vi "Nelson_Find_Whale_Color_Updated_Again.vi"(3 "error in":errorcluster, 5 "Image In":T1(plugin-control)) -> (0 "error out":errorcluster, 1 "Calibrated Centroid (Centroid 1)":cluster{"X Centroid":sgl, "Y Centroid":sgl} {"Y Centroid" format="%.2f"; "X Centroid" format="%.2f"}, 2 "Image Out":T1(plugin-control))   [LabVIEW 2014]
uses:
  <vilib>/vision/NI_Vision_Development_Module.lvlib
panel:
  out "Centroid (Centroid 1)":cluster{"X Centroid":sgl, "Y Centroid":sgl} {"Y Centroid" format="%.2f"; "X Centroid" format="%.2f"}
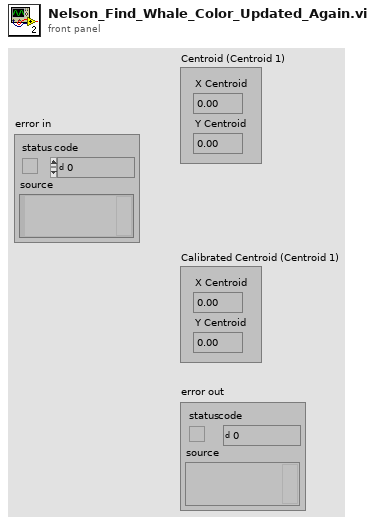
[diagram p1: front panel]
types:
  T1 = typedef "IMAQ Image.ctl" = refnum<image>
  T2 = cluster{"Global Rectangle":i32[], "Contours":cluster{"ID":enum32{"External", "Internal"}, "Type":u32, "Coordinates":i32[]}[]}
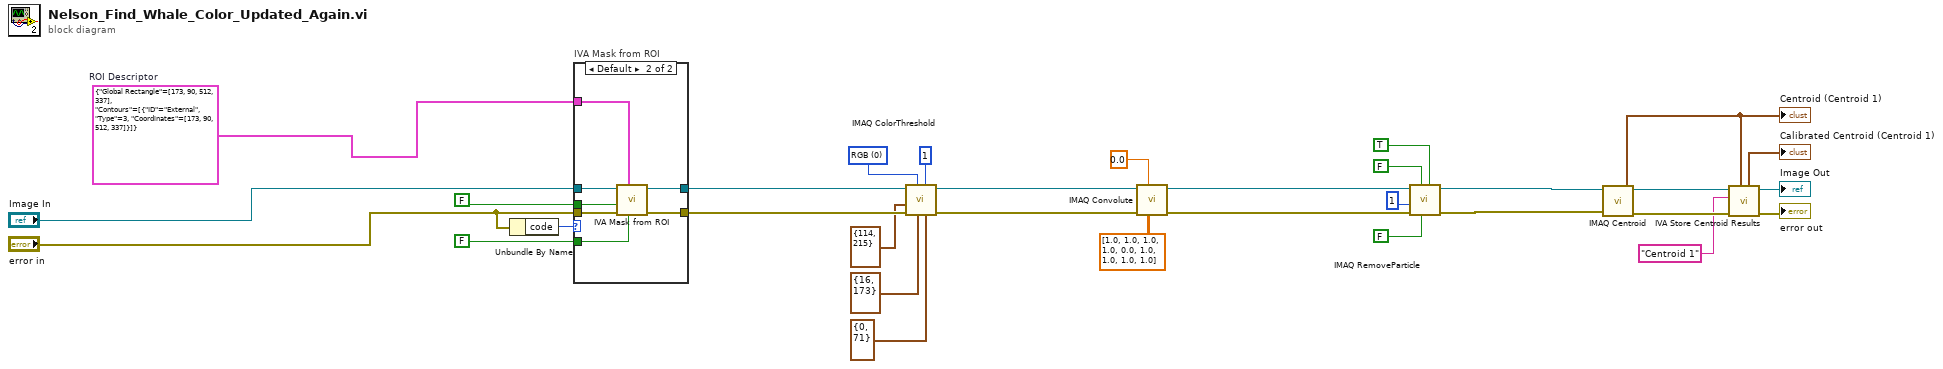
[diagram p0: block diagram]
diagram:
  w23 = u16 0 items=["RGB", "HSL", "HSV", "HSI"] ("Color Mode")
  w30 = T2 {"Global Rectangle"=[173, 90, 512, 337], "Contours"=[{"ID"=enum."External", "Type"=3, "Coordinates"=[173, 90, 512, 337]}]}  # ROI Descriptor
  n1 = Unbundle By Name("error in") -> ("code"=w25:i32)
  n2 = case "IVA Mask from ROI" shown="Default" w25 {
    tunnel: w30 -> [_ w39]
    tunnel: FALSE ("Shrink") -> [_ w38]
    tunnel: "Image In" -> [w32 w37]
    tunnel: "error in" -> [_ w36]
    tunnel: [_ w35] -> w27
    tunnel: [w32 w34] -> w19
    tunnel: FALSE ("Out / In") -> [_ w33]
    frame -1074396199, -1074396198 {
      # "Discard\nCoordinate\nSystem\nError"
    }
    frame Default {
      n3 = call <vilib>:"IVA Mask from ROI.vi"("Shrink"=w38, "ROI Descriptor"=w39, "error in (no error)"=w36, "Out / In"=w33, "Image Src"=w37) -> ("error out"=w35:errorcluster, "Image Out"=w34:T1)  [unwired: 5 out]
    }
  }
  n4 = call "IMAQ ColorThreshold"("Blue or Luma or Val or Inten Range"=cluster{"Lower value":i32, "Upper value":i32} {"Lower value"=0, "Upper value"=71}, "Replace Value"=1, "Green or Sat Range"=cluster{"Lower value":i32, "Upper value":i32} {"Lower value"=16, "Upper value"=173}, "Color Mode"=w23, "error in (no error)"=w27, "Red or Hue Range"=cluster{"Lower value":i32, "Upper value":i32} {"Lower value"=114, "Upper value"=215}, "Image Src"=w19) -> ("error out"=w18:errorcluster, "Image Dst Out"=w16:T1)  [unwired: 1 in, 2 out]
  n5 = call "IMAQ Convolute"("Kernel"=sgl[][] [[1.0, 1.0, 1.0], [1.0, 0.0, 1.0], [1.0, 1.0, 1.0]], "Divider (kernel sum)"=sgl 0.0 ("Divider"), "error in (no error)"=w18, "Image Src"=w16) -> ("error out"=w15:errorcluster, "Image Dst Out"=w9:T1)  [unwired: 3 in, 3 out]
  n6 = call "IMAQ RemoveParticle"("Connectivity 4/8 (8)"=TRUE, "Low Pass/High Pass (Low)"=FALSE, "Square/Hexa (Square)"=FALSE, "error in (no error)"=w15, "Number of Erosion"=1, "Image Src"=w9) -> ("error out"=w8:errorcluster, "Image Dst Out"=w5:T1)  [unwired: 1 in, 3 out]
  n7 = call "IMAQ Centroid"("error in (no error)"=w8, "Image"=w5) -> ("error out"=w7:errorcluster, "Centroid"=w2:cluster{"X Centroid":sgl, "Y Centroid":sgl})  [unwired: 1 in, 1 out]
  "Centroid (Centroid 1)" <- w2
  n8 = call <vilib>:"IVA Store Centroid Results.vi"("Centroid in"=w2, "error in (no error)"=w7, "Step Name"="Centroid 1", "Image in"=w5) -> ("error out"=→"error out":errorcluster, "Image dup"=→"Image Out":T1, "Calibrated Centroid"=→"Calibrated Centroid (Centroid 1)":cluster{"X":sgl, "Y":sgl})  [unwired: 5 out]
